vi "Read Labels.vi"(8 "error in (no error)":errorcluster, 10 "INI File Path":path, 11 "Control Info in":refnum<class "Control Info.lvclass">) -> (0 "error out":errorcluster, 2 "Labels [Additional Labels]":string[](array[string]), 3 "Control Info out":refnum<class "Control Info.lvclass">)   [LabVIEW 2017, in "Localization.lvlib" / "Control Info.lvclass"]
doc: "Reads the Labels that name the additional label options from the INI file. also reads the VI Path from the INI file and stores all that information into the class data.\n\nChoose Movement Consulting, LLC"
uses:
  Control Info.lvclass
  Control Info.lvclass/Control Info.ctl
  <vilib>/Utility/config.llb/Read Key (Path).vi
  <vilib>/Utility/config.llb/Read Key (String).vi
  <vilib>/Utility/config.llb/NI_LVConfig.lvlib
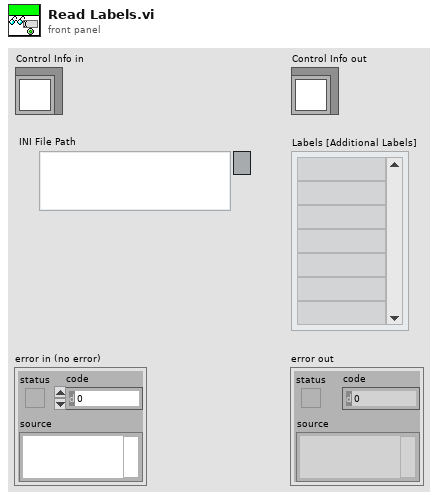
[diagram p1: front panel]
types:
  T1 = typedef "NI_LVConfig.lvlib/Config Data RefNum.ctl" = refnum<k1>
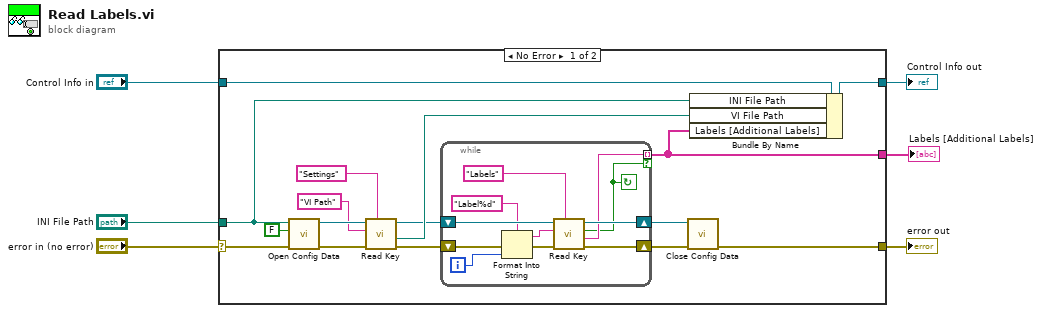
[diagram p0: block diagram]
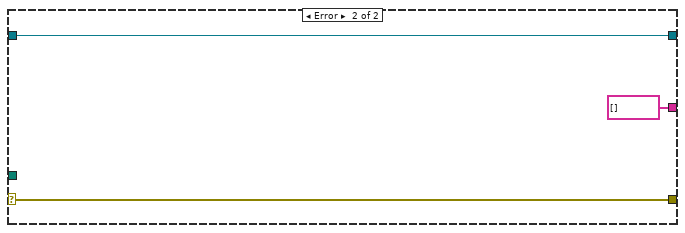
[diagram p2: hidden frame]
diagram:
  n1 = case shown="No Error" "error in (no error)" {
    selector: "error in (no error)" -> [w21 w36]
    tunnel: [w8 w36] -> w5
    tunnel: [w19 w35] -> w3
    tunnel: "Control Info in" -> [w22 w35]
    tunnel: "INI File Path" -> [w16 _]
    tunnel: [w9 string[] []] -> w1
    frame No Error {
      n2 = call <vilib>:"Open Config Data.vi"("error in (no error)"=w21, "create file if necessary (T)"=FALSE, "configuration file path"=w16) -> ("error out"=w17:errorcluster, "refnum"=w18:T1)  [unwired: 6 in, 1 out]
      n3 = call-poly <vilib>:"Read Key.vi"("section"="Settings", "error in (no error)"=w17, "key"="VI Path" ("section"), "refnum"=w18) -> ("error out"=w11:errorcluster, "value"=w13:path, "refnum out"=w12:T1)  [unwired: 4 in, 1 out]
      n4 = while {
        shift-right: [w31] -> w10
        shift-left: w11 -> [w29]
        shift-right: [w30] -> w7
        shift-left: w12 -> [w33]
        tunnel: [w24] -> w9 mode=indexing if=w23
        i -> [w27]
        stop <- w23 continue-if-true
        n5 = Format Into String(format string="Label%d" ("section"), error in=w29, w27) -> (resulting string=w25:string, error out=w28:errorcluster)  [unwired: 1 in]
        n6 = call-poly <vilib>:"Read Key.vi"("section"="Labels", "error in (no error)"=w28, "key"=w25, "refnum"=w33) -> ("error out"=w31:errorcluster, "value"=w24:string, "found?"=w23:bool, "refnum out"=w30:T1)  [unwired: 4 in]
      }
      n7 = call <vilib>:"Close Config Data.vi"("error in (no error)"=w10, "refnum"=w7) -> ("error out"=w8:errorcluster)  [unwired: 8 in, 1 out]
      n8 = Bundle By Name(cluster=w22, "INI File Path"=w16, "VI File Path"=w13, "Labels [Additional Labels]"=w9) -> (w19:refnum<class "Control Info.lvclass">)
    }
    frame Error {
    }
  }
  "error out" <- w5
  "Control Info out" <- w3
  "Labels [Additional Labels]" <- w1
